vi "Netburner_RD.vi"(0 "VISA resource name (COM Port #)":refnum<visa-resource-name>="COM3", 2 "Mode (0)":i32, 3 "Error In (no error)":errorcluster, 4 "Wait (sec)":dbl=0.25) -> (1 "Number of Bytes Received":u32, 5 "Return String from Device":string="\n\r", 6 "Error Out":errorcluster={"status"=FALSE, "code"=1073676294, "source"="VISA Read in Galvant_GPIB_Sample.vi"})   [LabVIEW 2013]
uses:
  Instance           3 34Saved   Prologix LabVIEW 7 Example .vi
  <vilib>/Instr/_visa.llb/VISA Configure Serial Port (Instr).vi
panel:
  out "Examples":string="Useful strings:\n+test\n+a:10\nID?"
  # "Netburner Read VI"
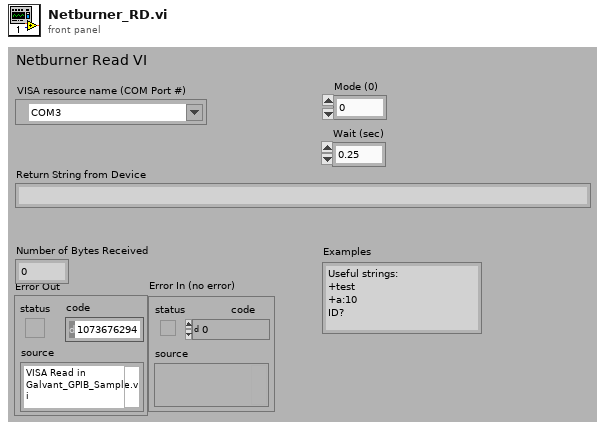
[diagram p1: front panel]
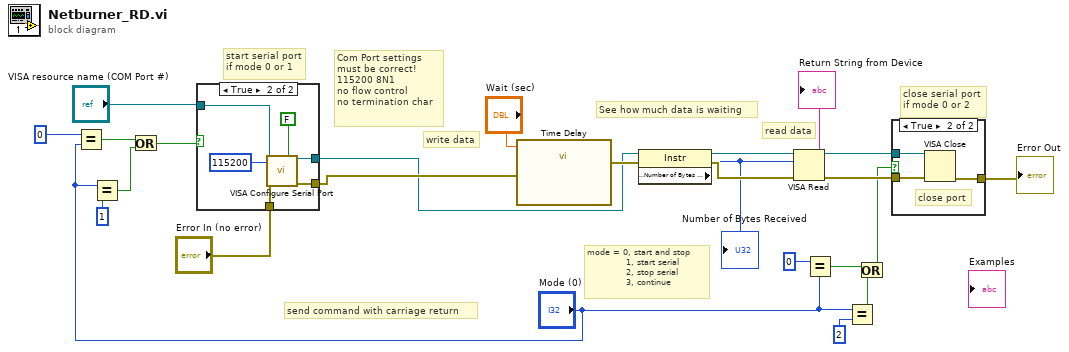
[diagram p0: block diagram]
diagram:
  # "write data"
  # "mode = 0, start and stop\n             1, start serial\n             2, stop serial\n             3, continue"
  # "Com Port settings\nmust be correct!\n115200 8N1\nno flow control\nno termination char"
  # "close serial port\nif mode 0 or 2"
  # "read data"
  # "See how much data is waiting"
  # "send command with carriage return"
  # "start serial port\nif mode 0 or 1"
  n1 = Equal?(x=0, y="Mode (0)") -> (x = y?=w7:bool)
  n2 = Equal?(x="Mode (0)", y=1) -> (x = y?=w5:bool)
  n3 = Or(x=w7, y=w5) -> (x .or. y?=w6:bool)
  n4 = case shown="True" w6 {
    tunnel: "VISA resource name (COM Port #)" -> [w26 w32]
    tunnel: [w26 w31] -> w1
    tunnel: [w25 w30] -> w2
    tunnel: "Error In (no error)" -> [w25 w27]
    frame False {
    }
    frame True {
      n5 = call-poly "VISA Configure Serial Port"("VISA resource name"=w32, "Enable Termination\nChar (T)"=FALSE, "baud rate (9600)"=115200, "error in (no error)"=w27) -> ("VISA resource name out"=w31:refnum<visa-resource-name>, "error out"=w30:errorcluster)  [unwired: 10 in]
    }
  }
  n6 = call "Time Delay"("error in (no error)"=w2, "Delay Time (s)"="Wait (sec)") -> ("error out"=w18:errorcluster)  [unwired: 9 in]
  n7 = property class="Instr"(reference=w1, error in=w18) -> (reference out=w16:refnum<visa-resource-name>, error out=w17:errorcluster, "Serial Settings:Number of Bytes at Serial Port"=w15:u32)
  "Number of Bytes Received" <- w15
  n8 = VISA Read(VISA resource name=w16, byte count=w15, error in (no error)=w17) -> (VISA resource name out=w23:refnum<visa-resource-name>, read buffer=→"Return String from Device":string, error out=w22:errorcluster)  [unwired: 1 out]
  n9 = Equal?(x=0, y="Mode (0)") -> (x = y?=w11:bool)
  n10 = Equal?(x="Mode (0)", y=2) -> (x = y?=w9:bool)
  n11 = Or(x=w11, y=w9) -> (x .or. y?=w8:bool)
  n12 = case shown="True" w8 {
    tunnel: w23 -> [_ w36]
    tunnel: w22 -> [w33 w35]
    tunnel: [w33 w34] -> w20
    frame False {
    }
    frame True {
      # "close port"
      n13 = VISA Close(VISA resource name=w36, error in (no error)=w35) -> (error out=w34:errorcluster)
    }
  }
  "Error Out" <- w20
